vi "PH_PILS.set Doors ExtExp.vi"(0 "i ref in":refnum<vi>, 5 "error in":errorcluster) -> (14 "i ref out":refnum<vi>, 19 "error out":errorcluster)   [LabVIEW 2014, in "PH_PILS.lvlib"]
doc: "This VI sets the GUI elements related to the doors at the external experiments."
uses:
  PH_PILS.lvlib
  PH_Basics/PH_Common/PH_Common.lvlib
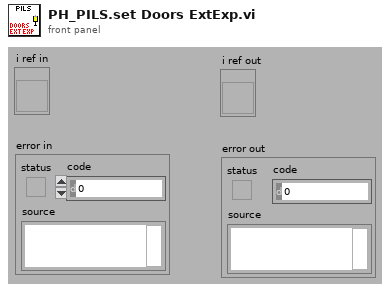
[diagram p1: front panel]
types:
  T1 = enum16{"unknown", "intern", "4 (Z6)", "3", "2", "1"}[]
  T2 = typedef "PH_PILS.lvlib/PH_PILS.i attribute.ctl" = cluster{"Boolean":cluster{"GUI Ref":refnum<vi>, "Status":i32}[], "GUI Refs Exp. Shutters":cluster{"1":refnum<vi>, "2":refnum<vi>, "3":refnum<vi>, "4":refnum<vi>}, "Tristate2Run GUI Refs":refnum<vi>[], "EO-Likes":cluster{"GUI Ref":refnum<vi>, "Status":i32}[], "Operation Mode":cluster{"Operation Mode":T3, "GUI":cluster{"Ref State":refnum<vi>, "Ref":refnum<vi>}, "Servicemode":cluster{"Tagname":string, "Status":i32}, "Labormode":cluster{"Tagname":string, "Status":i32}, "Searchmode":cluster{"Tagname":string, "Status":i32}, "Shotmode":cluster{"Tagname":string, "Status":i32}}, "Submode":cluster{"Submode":T4, "GUI":cluster{"Ref State":refnum<vi>, "Ref":refnum<vi>}, "Submode":cluster{"Tagname":string, "Status":i32}}, "Experiment":cluster{"Experiment":enum16{"unknown", "intern", "4 (Z6)", "3", "2", "1"}, "GUI":cluster{"Ref State":refnum<vi>, "Ref":refnum<vi>}, "intern":cluster{"Tagname":string, "Status":i32}, "Exp 4":cluster{"Tagname":string, "Status":i32}, "Exp 3":cluster{"Tagname":string, "Status":i32}, "Exp 2":cluster{"Tagname":string, "Status":i32}, "Exp 1":cluster{"Tagname":string, "Status":i32}}, "TristateNormal":cluster{"GUI Ref":refnum<vi>, "Status":i32}[], "Door Tags":cluster{"GUI Ref":refnum<vi>, "Status":i32}[], "GUIlessTags":cluster{"Name":string, "Status":i32}[], "Beamline GUI Refs":refnum<vi>[], "Special Boolean":cluster{"GUI Ref":refnum<vi>, "Status":i32}[], "Laserpower":cluster{"GUI Ref":refnum<vi>, "Status":i32}[], "Shutter":cluster{"GUI Ref":refnum<vi>, "Status":i32}[], "Tristate EO Like":cluster{"GUI Ref":refnum<vi>, "Status":i32}[], "PP":cluster{"GUI Ref":refnum<vi>, "Status":i32, "Head Ref":refnum<vi>, "Slider Ref":refnum<vi>}[], "Switch Knobs":cluster{"GUI Ref":refnum<vi>, "Status":i32}[], "Latch Knob GUI Refs":refnum<vi>[], "FailureCounter":i32, "Enabled Status":cluster{"Laser":i32, "PreAmp":i32, "MainAmp":i32}, "Mercury":refnum<vi>, "Instance Rods":string, "Logfile":path, "Beckhoff-Instance Internal":string, "Beckhoff-Instance External":string, "Enabling Rights":cluster{"Name":string, "Password":string, "PA?":bool, "MA?":bool, "Exp?":bool}[]}
  T3 = typedef "PH_PILS.lvlib/PH_PILS.Operation Mode.ctl" = enum16{"unknown", "Service", "Labor", "Search", "Shot"}
  T4 = typedef "PH_PILS.lvlib/PH_PILS.Submode.ctl" = enum16{"unknown", "HV-Normal", "HV-Test"}
  T5 = enum16{"unknown", "intern", "4 (Z6)", "3", "2", "1"}
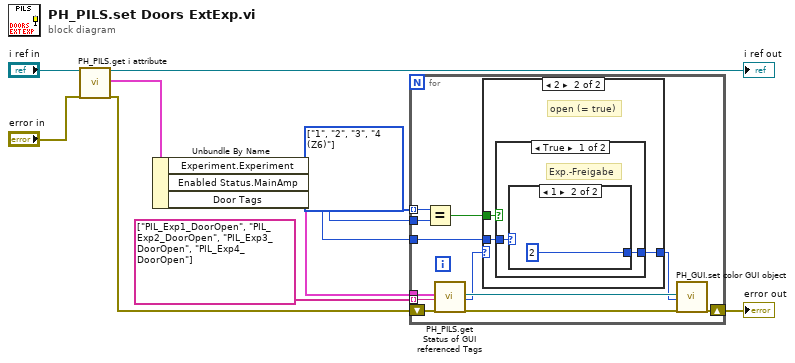
[diagram p0: block diagram]
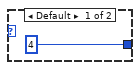
[diagram p3: hidden frame]
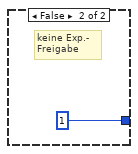
[diagram p4: hidden frame]
diagram:
  w2 = T1 [enum."1", enum."2", enum."3", enum."4 (Z6)"] items=["unknown", "intern", "4 (Z6)", "3", "2", "1"]
  n1 = call "PH_PILS.get i attribute.vi"("i ref in"="i ref in", "error in (no error)"="error in") -> ("i ref out"=→"i ref out":refnum<vi>, "i attribute"=w8:T2, "error out"=w4:errorcluster)  [unwired: 15 in]
  n2 = Unbundle By Name(w8) -> ("Experiment.Experiment"=w3:T5, "Enabled Status.MainAmp"=w1:i32, "Door Tags"=w5:cluster{"GUI Ref":refnum<vi>, "Status":i32}[])
  n3 = for {
    tunnel: w5 -> [w23]
    tunnel: string[] ["PIL_Exp1_DoorOpen", "PIL_Exp2_DoorOpen", "PIL_Exp3_DoorOpen", "PIL_Exp4_DoorOpen"] -> [w20] mode=indexing
    shift-right: [w19] -> w7
    shift-left: w4 -> [w22]
    tunnel: w3 -> [w15]
    tunnel: w2 -> [w14] mode=indexing
    tunnel: w1 -> [w12]
    n4 = Equal?(x=w14, y=w15) -> (x = y?=w13:bool)
    n5 = call "PH_PILS.get Status of GUI referenced Tags.vi"("Tags"=w23, "Tagname"=w20, "error in"=w22) -> ("GUI Ref"=w18:refnum<vi>, "Status"=w17:i32, "error out"=w21:errorcluster)  [unwired: 13 in, 1 out]
    n6 = case shown="2" w17 {
      selector: w17 -> [w24 _]
      tunnel: [w24 w27] -> w16
      tunnel: w13 -> [_ w26]
      tunnel: w12 -> [_ w25]
      frame 0, Default {
        # "no info,\nclosed (= false)"
      }
      frame 2 {
        # "open (= true)"
        n7 = case shown="True" w26 {
          tunnel: [w29 1] -> w27
          tunnel: w25 -> [w28 _]
          frame True {
            # "Exp.-Freigabe"
            n8 = case shown="1" w28 {
              tunnel: [4 2] -> w29
              frame Default {
              }
              frame 1 {
              }
            }
          }
          frame False {
            # "keine Exp.-\nFreigabe"
          }
        }
      }
    }
    n9 = call "PH_GUI.set color GUI object.vi"("GUI object Ref"=w18, "State"=w16, "error in (no error)"=w21) -> ("error out"=w19:errorcluster)  [unwired: 16 in]
  }
  "error out" <- w7
